vi "EncodeDataFrame.vi"(8 "ErrorIn":errorcluster, 11 "Packet":T1) -> (0 "ErrorOut":errorcluster, 3 "Frame":string)   [LabVIEW 2016]
doc: "Encode data frame in order to get string from measument packets and other data associated during implementation.\n\nIf there is an arror during processing or at the input, VI ends execution and throws error."
uses:
  FallSensor/Packet.ctl
  FallSensor/Sample.ctl
  FallSensor/Reading.ctl
  FallSensor/ReadingUnits/AccelReadingUnit.ctl
  FallSensor/ReadingUnits/GyroReadingUnit.ctl
  DataFrame/DataFrameSection.ctl
  DataFrame/DataFrameSectionsLen.ctl
  DataFrame/DataFrameContext.ctl
  FallSensor/EventStatus.ctl
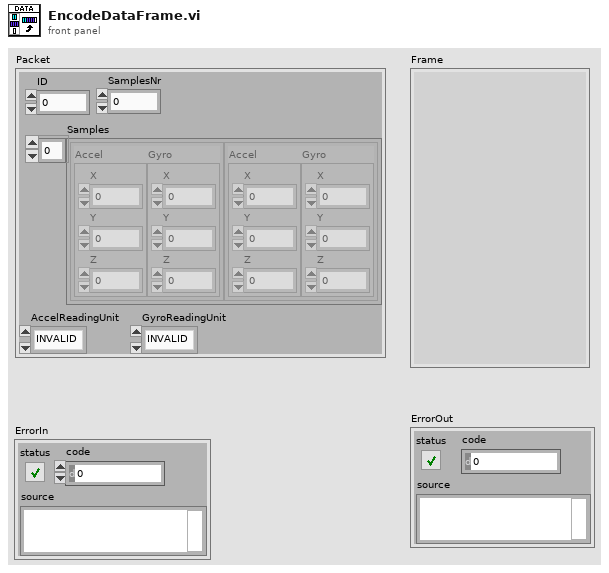
[diagram p1: front panel]
types:
  T1 = typedef "Packet.ctl" = cluster{"ID":u32, "SamplesNr":u32, "Samples":T2[], "AccelReadingUnit":T4, "GyroReadingUnit":T5}
  T2 = typedef "Sample.ctl" = cluster{"Accel":T3, "Gyro":T3}
  T3 = typedef "Reading.ctl" = cluster{"X":i16, "Y":i16, "Z":i16}
  T4 = typedef "AccelReadingUnit.ctl" = enum16{"INVALID", "RAW", "g"}
  T5 = typedef "GyroReadingUnit.ctl" = enum16{"INVALID", "RAW", "°/sec"}
  T6 = typedef "DataFrameContext.ctl" = cluster{"Frame":string, "FrameHeader":string, "FrameSectionsLen":T7, "Packets":T1[], "MeasFreq":u32, "EventStatus":T8, "PackedIDs":u32[]}
  T7 = typedef "DataFrameSectionsLen.ctl" = cluster{"Header":i32, "PacketID":i32, "Packet":i32, "Sample":i32}
  T8 = typedef "EventStatus.ctl" = enum16{"IDLE", "FALL", "NONE"}
  T9 = typedef "DataFrameSection.ctl" = enum16{"SOF", "Header", "PacketID", "Data", "EOF"}
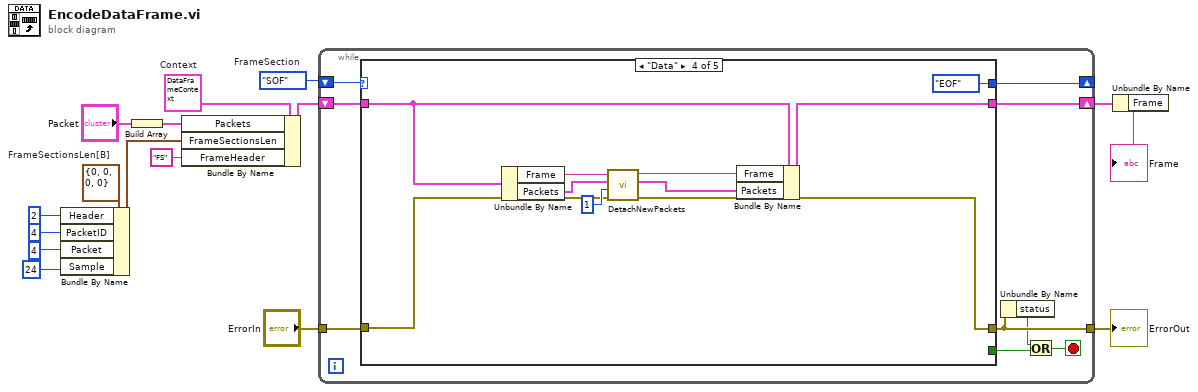
[diagram p0: block diagram]
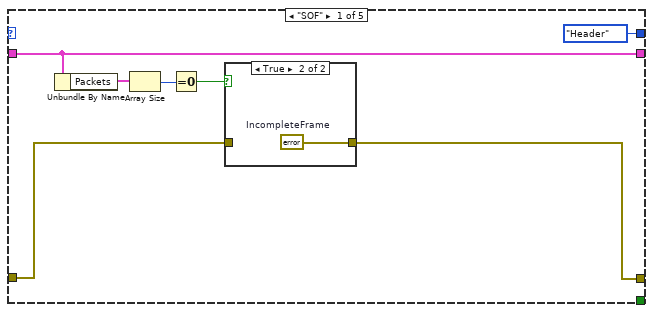
[diagram p2: hidden frame]
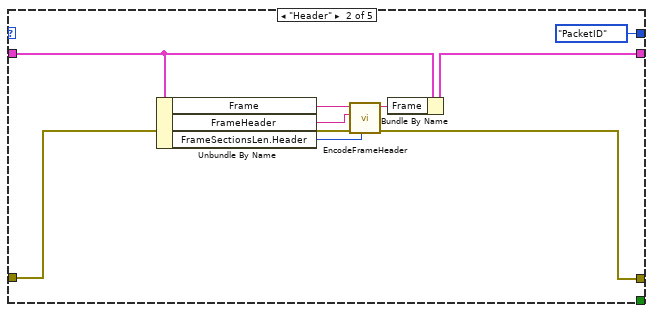
[diagram p4: hidden frame]
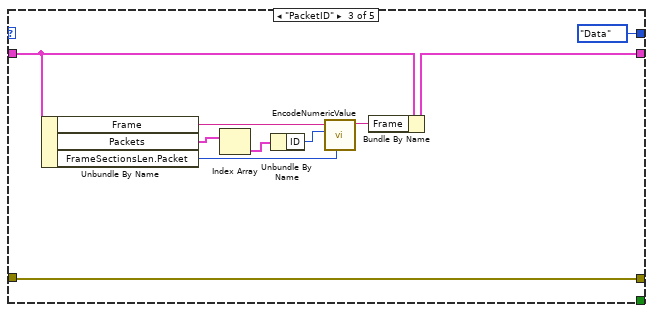
[diagram p5: hidden frame]
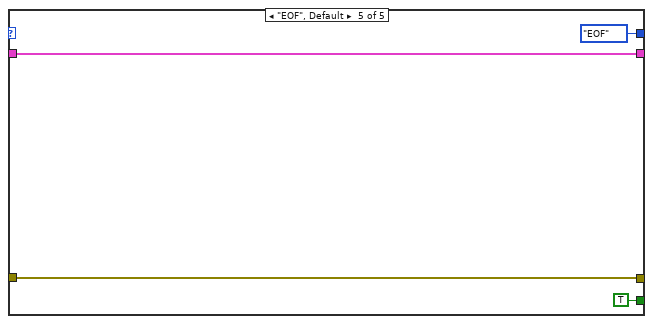
[diagram p6: hidden frame]
diagram:
  w14 = T6 {"Frame"="", "FrameHeader"="", "FrameSectionsLen"={"Header"=0, "PacketID"=0, "Packet"=0, "Sample"=0}, "Packets"=[], "MeasFreq"=0, "EventStatus"=enum."IDLE", "PackedIDs"=[]}  # Context
  w5 = T7 {"Header"=0, "PacketID"=0, "Packet"=0, "Sample"=0}  # FrameSectionsLen[B]
  w4 = DataFrameSection."SOF"  # FrameSection
  n1 = Bundle By Name(cluster=w5, "Header"=2, "PacketID"=4 ("PacketName"), "Packet"=4 ("Config"), "Sample"=24 ("Config")) -> (w12:T7)
  n2 = Build Array("Packet") -> (w1:T1[])
  n3 = Bundle By Name(cluster=w14, "Packets"=w1, "FrameSectionsLen"=w12, "FrameHeader"="FS") -> (w11:T6)
  n4 = while {
    shift-right: [w17] -> _
    shift-left: w4 -> [w18]
    tunnel: "ErrorIn" -> [w25]
    tunnel: [w22] -> w15
    shift-right: [w23] -> w10
    shift-left: w11 -> [w24]
    stop <- w21 stop-if-true
    n5 = case shown="\"Data\"" w18 {
      tunnel: w25 -> [w27 w40 w53 w55 w67]
      tunnel: [w26 w36 w53 w54 w67] -> w22
      tunnel: w24 -> [w31 w39 w47 w57 w65]
      tunnel: [w31 w38 w46 w56 w65] -> w23
      tunnel: [_ _ _ _ TRUE] -> w19
      tunnel: [DataFrameSection."Header" ("FrameSection") DataFrameSection."PacketID" ("FrameSection") DataFrameSection."Data" ("FrameSection") DataFrameSection."EOF" ("FrameSection") DataFrameSection."EOF" ("FrameSection")] -> w17
      frame "SOF" {
        n6 = Unbundle By Name(w31) -> ("Packets"=w30:T1[])
        n7 = Array Size(array=w30) -> (size(s)=w29:i32)
        n8 = Equal To 0?(x=w29) -> (x = 0?=w28:bool)
        n9 = case shown="True" w28 {
          tunnel: w27 -> [w33 _]
          tunnel: [w33 w34] -> w26
          frame False {
          }
          frame True {
            w34 = errorcluster {"status"=TRUE, "code"=1, "source"="Incomplete frame"}  # IncompleteFrame
          }
        }
      }
      frame "Header" {
        n10 = Unbundle By Name(w39) -> ("Frame"=w42:string, "FrameHeader"=w41:string, "FrameSectionsLen.Header"=w35:i32)
        n11 = call "EncodeFrameHeader.vi"("HeaderLen"=w35, "ErrorIn"=w40, "Header"=w41, "FrameIn"=w42) -> ("ErrorOut"=w36:errorcluster, "FrameOut"=w37:string)  [unwired: 6 in]
        n12 = Bundle By Name(cluster=w39, "Frame"=w37) -> (w38:T6)
      }
      frame "PacketID" {
        n13 = Unbundle By Name(w47) -> ("Frame"=w51:string, "Packets"=w49:T1[], "FrameSectionsLen.Packet"=w50:i32)
        n14 = Index Array(array=w49) -> (element=w45:T1)  [unwired: 1 in]
        n15 = Unbundle By Name(w45) -> ("ID"=w44:u32)
        n16 = call "EncodeNumericValue.vi"("DataLen"=w50, "NumericValue"=w44, "FrameIn"=w51) -> ("FrameOut"=w48:string)  [unwired: 8 in]
        n17 = Bundle By Name(cluster=w47, "Frame"=w48) -> (w46:T6)
      }
      frame "Data" {
        n18 = Unbundle By Name(w57) -> ("Frame"=w62:string, "Packets"=w61:T1[])
        n19 = call "DetachNewPackets.vi"("ErrorIn"=w55, "PacketsNum"=u32 1, "PacketsIn"=w61, "FrameIn"=w62) -> ("ErrorOut"=w54:errorcluster, "PacketsOut"=w58:T1[], "FrameOut"=w59:string)  [unwired: 5 in]
        n20 = Bundle By Name(cluster=w57, "Frame"=w59, "Packets"=w58) -> (w56:T6)
      }
      frame "EOF", Default {
      }
    }
    n21 = Unbundle By Name(w22) -> ("status"=w20:bool)
    n22 = Or(x=w20, y=w19) -> (x .or. y?=w21:bool)
  }
  "ErrorOut" <- w15
  n23 = Unbundle By Name(w10) -> ("Frame"=→"Frame":string)
